vi "WSVCAP SHL Host LL RFFE Write.vi"(0 "RTFFE Data [DUT Ordered]":u8[][](array[numeric]) format="%.0x", 1 "Wait Ticks":u32, 2 "Slave Address":u8, 5 "Socket Mask":u16=1 format="%02x", 7 "Cycle CMD Lengths Out (bits)":u8[](array[numeric]), 9 "Cycle CMD Delay Out (ticks)":u32[](array[numeric]), 11 "error in":errorcluster) -> (8 "Status":u8[](array[numeric]), 15 "error out":errorcluster)   [LabVIEW 2012]
uses:
  Type Defs/WSVCAP SHL Top Level Write Read State Enum.ctl
  Type Defs/WSVCAP SHL State.ctl
  Type Defs/WSVCAP SHL Top Level Control Enum.ctl
  Type Defs/WSVCAP SHL Transaction Enum.ctl
panel:
  out "Write Data":u64[](array[numeric]) format="%032b"
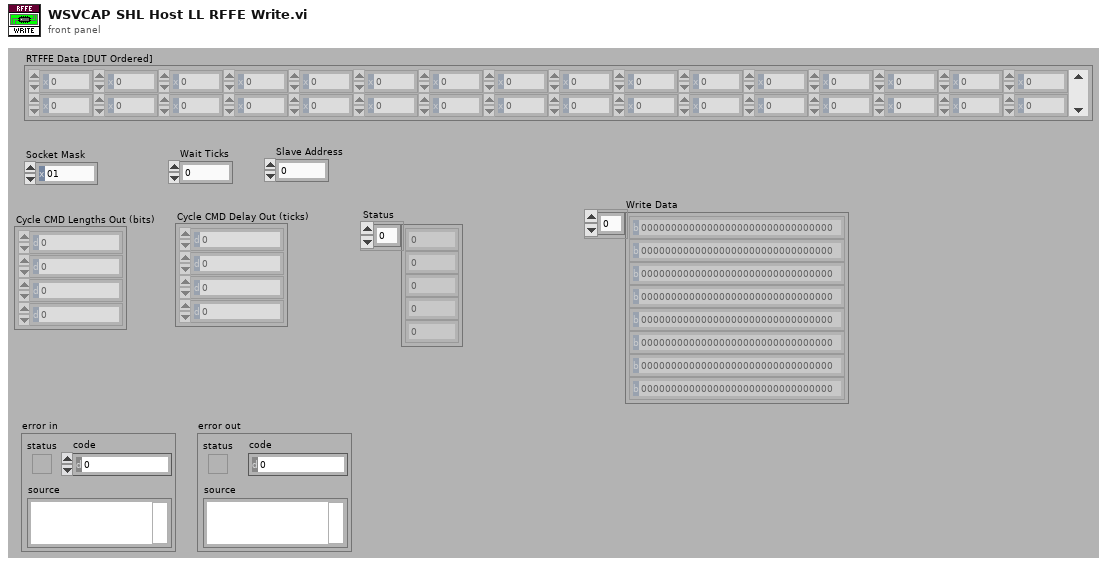
[diagram p1: front panel]
types:
  T1 = typedef "WSVCAP SHL Top Level Write Read State Enum.ctl" = enum16{"Start", "Write", "Read", "Get Status", "Wait Until Done"}
  T2 = typedef "WSVCAP SHL State.ctl" = enum8{"Idle", "Transfer Data"}
  T3 = typedef "WSVCAP SHL Transaction Enum.ctl" = enum16{"I2C-Read Data", "I2C-Write Data", "SPI-Write/Read Data", "RFFE-Ext Write", "RFFE-Ext Read"}
  T4 = typedef "WSVCAP SHL Top Level Control Enum.ctl" = enum16{"Start", "Cmd", "Transaction", "Wait Ticks", "Socket Mask", "Slave Address", "Sub Address", "Bytes to Write", "Bytes to Read", "Write Data", "Write Flag", "Read Data", "Read Flag", "Ack Read", "Read Status Flag", "Ack Read Status", "Status", "Cycle Count", "Stop Cycle", "Exit"}
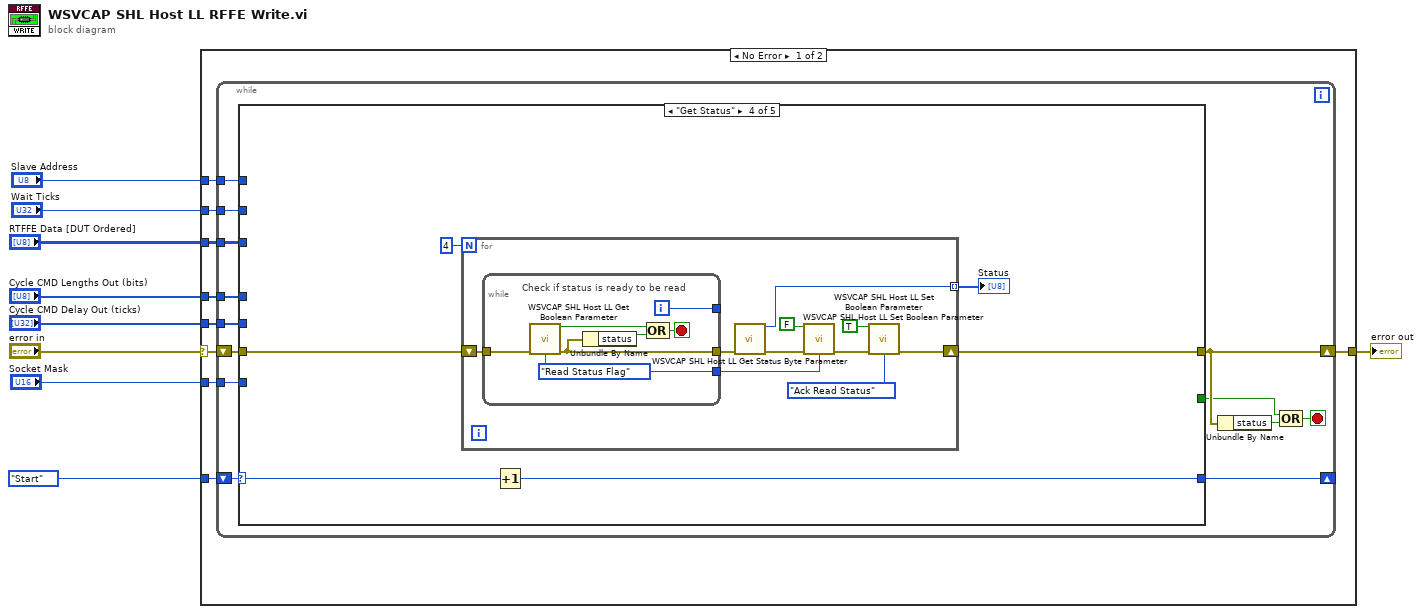
[diagram p0: block diagram]
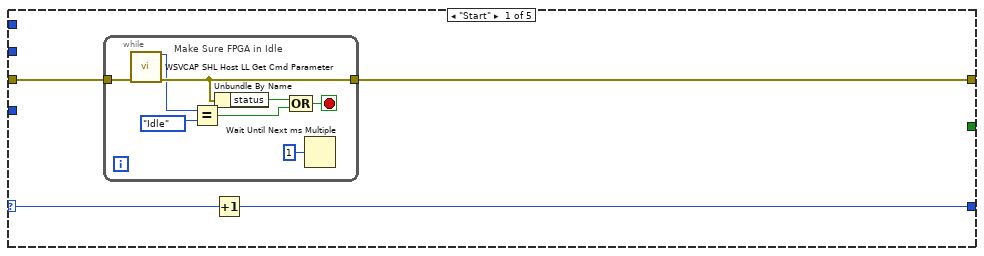
[diagram p2: hidden frame]
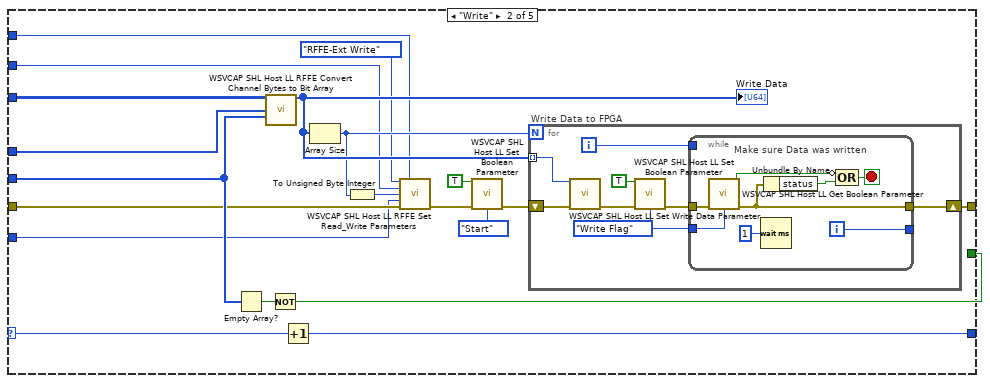
[diagram p3: hidden frame]
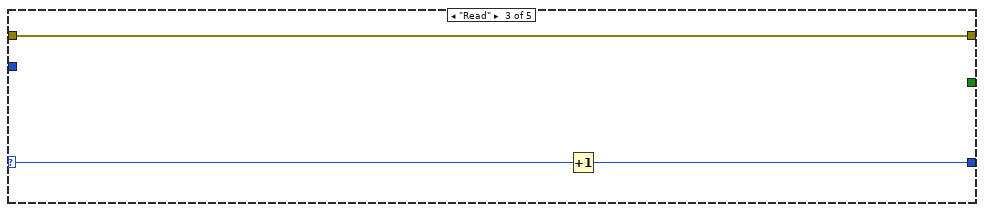
[diagram p4: hidden frame]
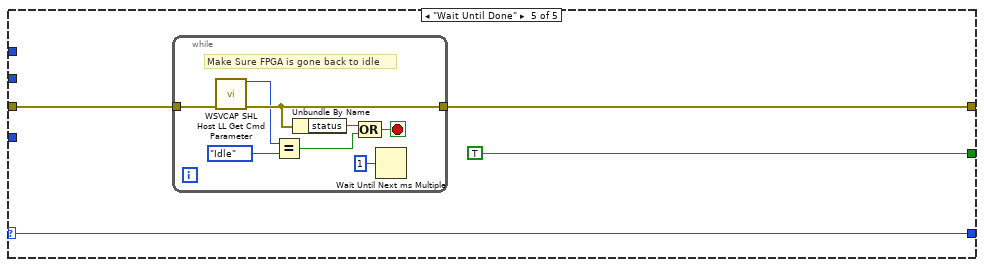
[diagram p5: hidden frame]
diagram:
  n1 = case shown="No Error" "error in" {
    selector: "error in" -> [w14 w118]
    tunnel: [w18 w118] -> w9
    tunnel: WSVCAP_SHL_Top_Level_Write_Read_State_Enum."Start" ("Write Read State") -> [w17 _]
    tunnel: "RTFFE Data [DUT Ordered]" -> [w16 _]
    tunnel: "Socket Mask" -> [w15 _]
    tunnel: "Cycle CMD Lengths Out (bits)" -> [w13 _]
    tunnel: "Cycle CMD Delay Out (ticks)" -> [w12 _]
    tunnel: "Wait Ticks" -> [w11 _]
    tunnel: "Slave Address" -> [w10 _]
    frame No Error {
      n2 = while {
        shift-right: [w30] -> w18
        shift-left: w14 -> [w31]
        shift-right: [w25] -> _
        shift-left: w17 -> [w26]
        tunnel: w16 -> [w24]
        tunnel: w15 -> [w23]
        tunnel: w13 -> [w22]
        tunnel: w12 -> [w21]
        tunnel: w11 -> [w20]
        tunnel: w10 -> [w19]
        stop <- w27 stop-if-true
        n3 = case shown="\"Get Status\"" w26 {
          selector: w26 -> [w34 w62 w82 w86 w107]
          tunnel: w31 -> [w35 w51 w80 w88 w109]
          tunnel: [w32 w63 w80 w87 w108] -> w30
          tunnel: [_ w56 _ _ TRUE] -> w29
          tunnel: [w33 w60 w81 w85 w107] -> w25
          tunnel: w24 -> [_ w47 _ _ _]
          tunnel: w23 -> [_ w48 _ _ _]
          tunnel: w22 -> [_ w59 _ _ _]
          tunnel: w21 -> [_ w58 _ _ _]
          tunnel: w20 -> [_ w46 _ _ _]
          tunnel: w19 -> [_ w44 _ _ _]
          frame "Start" {
            n4 = while {
              tunnel: w35 -> [w39]
              tunnel: [w38] -> w32
              stop <- w43 stop-if-true
              # "Make Sure FPGA in Idle"
              n5 = call "WSVCAP SHL Host LL Get Cmd Parameter.vi"("error in (no error)"=w39) -> ("I2C_Cmd"=w37:T2, "error out"=w38:errorcluster)  [unwired: 13 in]
              n6 = Equal?(x=w37, y=WSVCAP_SHL_State."Idle" ("Type")) -> (x = y?=w41:bool)
              n7 = Unbundle By Name(w38) -> ("status"=w36:bool)
              n8 = Compound Arithmetic op=OR(w36, w41) -> (w43:bool)
              n9 = Wait Until Next ms Multiple(millisecond multiple=u32 1) -> ()  [unwired: 1 out]
            }
            n10 = Increment(x=w34) -> (x+1=w33:T1)
          }
          frame "Write" {
            # "Write Data to FPGA"
            n11 = Empty Array?(array=w58) -> (empty?=w57:bool)
            n12 = call "WSVCAP SHL Host LL RFFE Convert Channel Bytes to Bit Array.vi"("RFFE Data [DUT Ordered]"=w47, "Cycle CMD Lengths Out (bits)"=w59, "Cycle CMD Delay Out (ticks)"=w58) -> ("Write Data"=w61:u64[])  [unwired: 12 in]
            "Write Data" <- w61
            n13 = Not(x=w57) -> (.not. x?=w56:bool)
            n14 = Increment(x=w62) -> (x+1=w60:T1)
            n15 = Array Size(array=w61) -> (size(s)=w49:i32)
            n16 = To Unsigned Byte Integer(number=w49) -> (unsigned 8bit integer=w52:u8)
            n17 = call "WSVCAP SHL Host LL RFFE Set Read_Write Parameters.vi"("Transaction"=WSVCAP_SHL_Transaction_Enum."RFFE-Ext Write", "Slave Address"=w44, "Wait Ticks"=w46, "Bytes to Write"=w52, "Socket Mask [U16]"=w48, "error in (no error)"=w51) -> ("error out"=w55:errorcluster)  [unwired: 9 in]
            n18 = call "WSVCAP SHL Host LL Set Boolean Parameter.vi"("Boolean In"=TRUE, "error in (no error)"=w55, "FPGA Top Level Control"=WSVCAP_SHL_Top_Level_Control_Enum."Start") -> ("error out"=w50:errorcluster)  [unwired: 12 in]
            n19 = for {
              N: w49 -> [_]
              shift-right: [w71] -> w63
              shift-left: w50 -> [w70]
              tunnel: w61 -> [w69] mode=indexing
              i -> [w64]
              w65 = WSVCAP_SHL_Top_Level_Control_Enum."Write Flag" ("FPGA Top Level Control")
              n20 = call "WSVCAP SHL Host LL Set Write Data Parameter.vi"("Write Byte In"=w69, "error in (no error)"=w70) -> ("error out"=w68:errorcluster)  [unwired: 13 in]
              n21 = call "WSVCAP SHL Host LL Set Boolean Parameter.vi"("Boolean In"=TRUE, "error in (no error)"=w68, "FPGA Top Level Control"=w65) -> ("error out"=w66:errorcluster)  [unwired: 12 in]
              n22 = while {
                tunnel: w66 -> [w77]
                tunnel: [w76] -> w71
                tunnel: w65 -> [w74]
                tunnel: w64 -> [_]
                tunnel: [w72] -> _
                i -> [w72]
                stop <- w79 stop-if-true
                # "Make sure Data was written"
                n23 = call "WSVCAP SHL Host LL Get Boolean Parameter.vi"("error in (no error)"=w77, "FPGA Top Level Control"=w74) -> ("Boolean Out"=w75:bool, "error out"=w76:errorcluster)  [unwired: 12 in]
                n24 = Wait (ms)(milliseconds to wait=u32 1) -> ()  [unwired: 1 out]
                n25 = Unbundle By Name(w76) -> ("status"=w73:bool)
                n26 = Compound Arithmetic op=OR(invert w75, w73) -> (w79:bool)
              }
            }
          }
          frame "Read" {
            n27 = Increment(x=w82) -> (x+1=w81:T1)
          }
          frame "Get Status" {
            n28 = for {
              N: 4 -> [_]
              shift-right: [w97] -> w87
              shift-left: w88 -> [w98]
              tunnel: [w89] -> w83 mode=indexing
              n29 = while {
                tunnel: w98 -> [w103]
                tunnel: [w102] -> w96
                tunnel: [w100] -> w94
                tunnel: [w99] -> _
                i -> [w99]
                stop <- w105 stop-if-true
                w100 = WSVCAP_SHL_Top_Level_Control_Enum."Read Status Flag" ("FPGA Top Level Control")
                # "Check if status is ready to be read"
                n30 = call "WSVCAP SHL Host LL Get Boolean Parameter.vi"("error in (no error)"=w103, "FPGA Top Level Control"=w100) -> ("Boolean Out"=w104:bool, "error out"=w102:errorcluster)  [unwired: 12 in]
                n31 = Unbundle By Name(w102) -> ("status"=w101:bool)
                n32 = Compound Arithmetic op=OR(w104, w101) -> (w105:bool)
              }
              n33 = call "WSVCAP SHL Host LL Get Status Byte Parameter.vi"("error in (no error)"=w96) -> ("I2C Status Byte"=w89:u8, "error out"=w95:errorcluster)  [unwired: 13 in]
              n34 = call "WSVCAP SHL Host LL Set Boolean Parameter.vi"("Boolean In"=FALSE ("Read Flag"), "error in (no error)"=w95, "FPGA Top Level Control"=w94) -> ("error out"=w90:errorcluster)  [unwired: 12 in]
              n35 = call "WSVCAP SHL Host LL Set Boolean Parameter.vi"("Boolean In"=TRUE ("Write Flag"), "error in (no error)"=w90, "FPGA Top Level Control"=WSVCAP_SHL_Top_Level_Control_Enum."Ack Read Status") -> ("error out"=w97:errorcluster)  [unwired: 12 in]
            }
            "Status" <- w83
            n36 = Increment(x=w86) -> (x+1=w85:T1)
          }
          frame "Wait Until Done" {
            n37 = while {
              tunnel: w109 -> [w112]
              tunnel: [w111] -> w108
              stop <- w114 stop-if-true
              # "Make Sure FPGA is gone back to idle"
              n38 = call "WSVCAP SHL Host LL Get Cmd Parameter.vi"("error in (no error)"=w112) -> ("I2C_Cmd"=w110:T2, "error out"=w111:errorcluster)  [unwired: 13 in]
              n39 = Equal?(x=w110, y=WSVCAP_SHL_State."Idle") -> (x = y?=w115:bool)
              n40 = Unbundle By Name(w111) -> ("status"=w116:bool)
              n41 = Compound Arithmetic op=OR(w116, w115) -> (w114:bool)
              n42 = Wait Until Next ms Multiple(millisecond multiple=u32 1) -> ()  [unwired: 1 out]
            }
          }
        }
        n43 = Unbundle By Name(w30) -> ("status"=w28:bool)
        n44 = Compound Arithmetic op=OR(w29, w28) -> (w27:bool)
      }
    }
    frame Error {
    }
  }
  "error out" <- w9
